vi "JSONDouble.vi"(9 "return":dbl) -> (3 "JSON string":string)   [LabVIEW 2026]
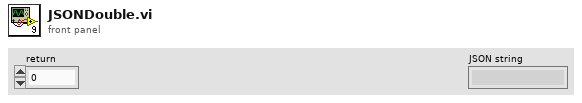
[diagram p1: front panel]
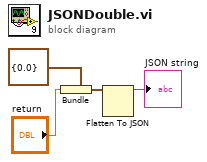
[diagram p0: block diagram]
diagram:
  n1 = Bundle(cluster=cluster{"return":dbl} {"return"=0.0}, "return"="return") -> (w4:cluster{"return":dbl})
  n2 = Flatten To JSON(anything=w4) -> (JSON string=→"JSON string":string)  [unwired: 2 in, 1 out]
